vi "读DS预定义数据项.vi"() -> ()   [LabVIEW 2010]
panel:
  out "数据3":bool
  out "数据2":string
  out "数据1":dbl
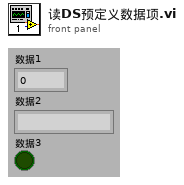
[diagram p1: front panel]
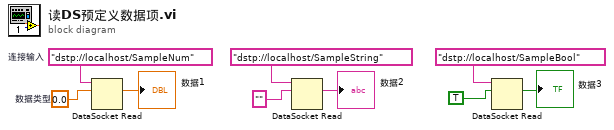
[diagram p0: block diagram]
diagram:
  w9 = 0.0  # 数据类型
  w1 = "dstp://localhost/SampleNum"  # 连接输入
  n1 = DataSocket Read ("读取DataSocket")(10:w9, 11:w1) -> (2:→"数据1":dbl)  [unwired: 3 in, 6 out]
  n2 = DataSocket Read(10:"", 11:"dstp://localhost/SampleString" ("connection in")) -> (2:→"数据2":string)  [unwired: 3 in, 6 out]
  n3 = DataSocket Read(10:TRUE, 11:"dstp://localhost/SampleBool" ("connection in")) -> (2:→"数据3":bool)  [unwired: 3 in, 6 out]
